vi "ZoneVacuumCtrl.vi"(7 "DecimalIn":u8, 8 "Error In":errorcluster, 9 "Position":enum16{"1", "2"}(ring), 10 "Zone":enum16{"ZoneA", "ZoneB", "ZoneC", "ZoneD"}(ring), 11 "ControlType":T2(ring)=enum."DecimalSwitch") -> (0 "Error Out":errorcluster, 2 "DecimalOut":u32, 3 "DecimalExpected":u32)   [LabVIEW 2019]
panel:
  out "GHTool":bool
  out "GHPlate":bool
  in  "Switches":T1
  out "BPTray":bool
  out "SiPCBTray":bool
  out "PUT1":bool
  out "SiPCB1":bool
  out "PUT2":bool
  out "SiPCB2":bool
  # "Zone control"
  # "ZoneA Indicator"
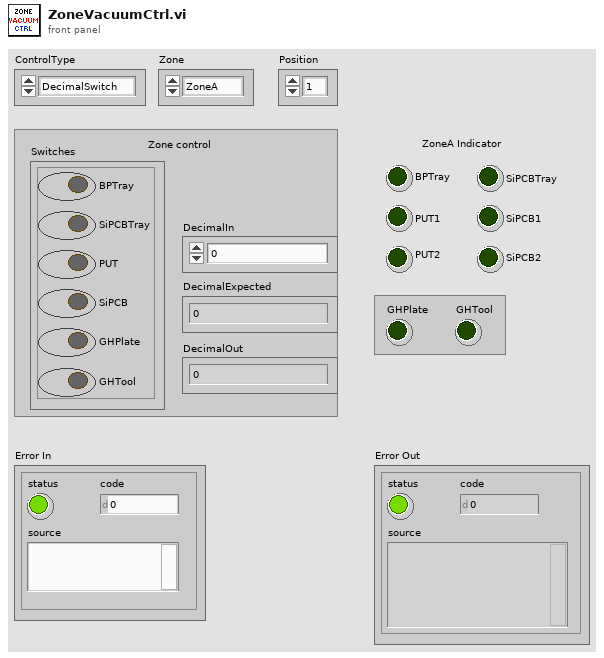
[diagram p1: front panel]
types:
  T1 = cluster{"BPTray":bool, "SiPCBTray":bool, "PUT":bool, "SiPCB":bool, "GHPlate":bool, "GHTool":bool}
  T2 = enum16{"BinarySwitch", "DecimalSwitch", "Conversion"}
  T3 = cluster{"data[0]":bool, "data[1]":bool, "data[2]":bool, "data[3]":bool, "data[4]":bool, "data[5]":bool, "data[6]":bool, "data[7]":bool, "data[8]":bool}
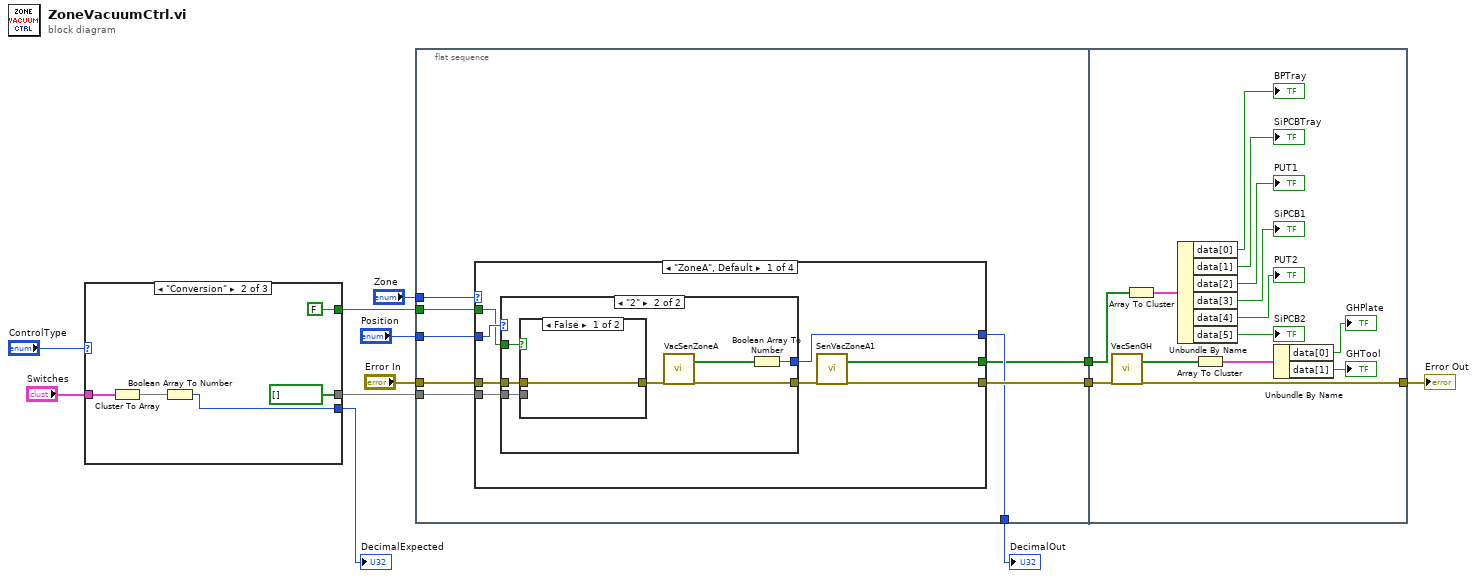
[diagram p0: block diagram]
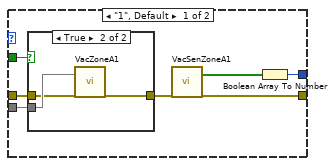
[diagram p2: hidden frame]
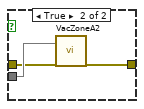
[diagram p4: hidden frame]
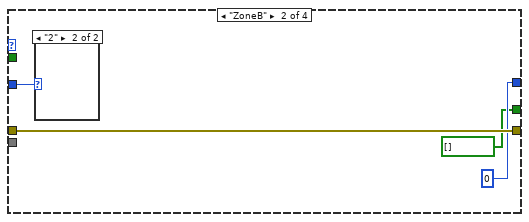
[diagram p5: hidden frame]
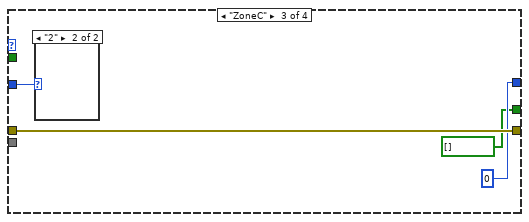
[diagram p7: hidden frame]
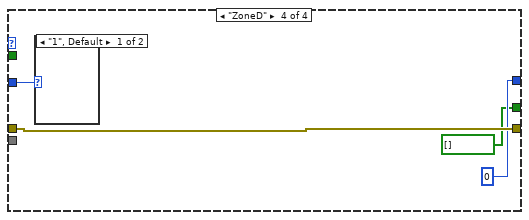
[diagram p9: hidden frame]
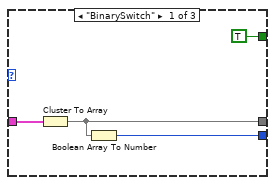
[diagram p11: hidden frame]
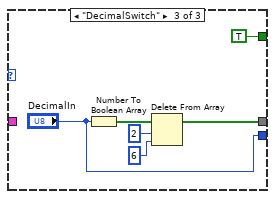
[diagram p12: hidden frame]
diagram:
  n1 = case shown="\"Conversion\"" "ControlType" {
    tunnel: [w15 bool[] [] ("Boolean array") w24] -> w10
    tunnel: [TRUE FALSE TRUE] -> w7
    tunnel: [w14 w19 "DecimalIn"] -> w6
    tunnel: "Switches" -> [w13 w17 _]
    frame "BinarySwitch" {
      n2 = Cluster To Array(cluster=w13) -> (array=w15:bool[])
      n3 = Boolean Array To Number(Boolean array=w15) -> (number=w14:u32)
    }
    frame "Conversion" {
      n4 = Cluster To Array(cluster=w17) -> (array=w18:bool[])
      n5 = Boolean Array To Number(Boolean array=w18) -> (number=w19:u32)
    }
    frame "DecimalSwitch" {
      n6 = Number To Boolean Array(number="DecimalIn") -> (Boolean array=w25:bool[])
      n7 = Delete From Array(array=w25, length=2, index=6) -> (array with subset deleted=w24:bool[])  [unwired: 1 out]
    }
  }
  "DecimalExpected" <- w6
  n8 = flat-sequence {
    tunnel: "Zone" -> [w35]
    tunnel: "Position" -> [w34]
    tunnel: w10 -> [w33]
    tunnel: "Error In" -> [w32]
    tunnel: w7 -> [w29]
    tunnel: [w31] -> w4
    tunnel: [w30] -> w3
    tunnel: [w28] -> w2
    tunnel: w4 -> [w83]
    tunnel: w2 -> [w84]
    tunnel: [w82] -> w1
    frame #0 {
      n9 = case shown="\"ZoneA\", Default" w35 {
        tunnel: w34 -> [w43 w69 w73 w77]
        tunnel: w33 -> [w42 _ _ _]
        tunnel: w32 -> [w41 w68 w72 w76]
        tunnel: [w36 w68 w72 w76] -> w31
        tunnel: [w40 u32 0 u32 0 u32 0] -> w30
        tunnel: w29 -> [w39 _ _ _]
        tunnel: [w38 bool[] [] ("data") bool[] [] ("data") bool[] [] ("data")] -> w28
        frame "ZoneA", Default {
          n10 = case shown="\"2\"" w43 {
            tunnel: w42 -> [w50 w61]
            tunnel: w41 -> [w49 w55]
            tunnel: [w48 w57] -> w37
            tunnel: [w46 w59] -> w40
            tunnel: w39 -> [w44 w56]
            frame "1", Default {
              n11 = case shown="True" w44 {
                tunnel: w50 -> [_ w54]
                tunnel: w49 -> [w51 w53]
                tunnel: [w51 w52] -> w47
                frame False {
                }
                frame True {
                  n12 = call "VacZoneA1"("data"=w54, "error in"=w53) -> ("error out"=w52:errorcluster)  [unwired: 16 in, 1 out]
                }
              }
              n13 = call "VacSenZoneA1"("error in"=w47) -> ("data"=w45:bool[], "error out"=w48:errorcluster)  [unwired: 16 in, 1 out]
              n14 = Boolean Array To Number(Boolean array=w45) -> (number=w46:u32)
            }
            frame "2" {
              n15 = case shown="False" w56 {
                tunnel: w61 -> [_ w65]
                tunnel: [w62 w64] -> w58
                tunnel: w55 -> [w62 w63]
                frame False {
                }
                frame True {
                  n16 = call "VacZoneA2"("data"=w65, "error in"=w63) -> ("error out"=w64:errorcluster)  [unwired: 16 in, 1 out]
                }
              }
              n17 = call "VacSenZoneA"("error in"=w58) -> ("data"=w60:bool[], "error out"=w57:errorcluster)  [unwired: 16 in, 1 out]
              n18 = Boolean Array To Number(Boolean array=w60) -> (number=w59:u32)
            }
          }
          n19 = call "SenVacZoneA1"("error in"=w37) -> ("data"=w38:bool[], "error out"=w36:errorcluster)  [unwired: 16 in, 1 out]
        }
        frame "ZoneB" {
          n20 = case shown="\"2\"" w69 {
            frame "1", Default {
            }
            frame "2" {
            }
          }
        }
        frame "ZoneC" {
          n21 = case shown="\"2\"" w73 {
            frame "1", Default {
            }
            frame "2" {
            }
          }
        }
        frame "ZoneD" {
          n22 = case shown="\"1\", Default" w77 {
            frame "1", Default {
            }
            frame "2" {
            }
          }
        }
      }
    }
    frame #1 {
      n23 = call "VacSenGH"("error in"=w83) -> ("data"=w81:bool[], "error out"=w82:errorcluster)  [unwired: 16 in, 1 out]
      n24 = Array To Cluster(array=w84) -> (cluster=w91:T3)
      n25 = Unbundle By Name(w91) -> ("data[0]"=→"BPTray":bool, "data[1]"=→"SiPCBTray":bool, "data[2]"=→"PUT1":bool, "data[3]"=→"SiPCB1":bool, "data[4]"=→"PUT2":bool, "data[5]"=→"SiPCB2":bool)
      n26 = Array To Cluster(array=w81) -> (cluster=w80:T3)
      n27 = Unbundle By Name(w80) -> ("data[0]"=→"GHPlate":bool, "data[1]"=→"GHTool":bool)
    }
  }
  "Error Out" <- w1
  "DecimalOut" <- w3
